vi "Plot Polar Datab.vi"(4 "polar attributes":T3={"maximum"=0.011811645350765643, "minimum"=0.0, "clip to min"=FALSE, "log"=FALSE, "grid color"=6710886, "plot color"=4456703, "fmt and prec"={"format"=enum."Decimal", "precision"=1}, "visible section"=8} {"minimum" format="%.2f"; "maximum" format="%.2f"}, 5 "grid measurements":T2={"pixel center"={"x"=350, "y"=350}, "scale factors"={"a"=28023.191534322883, "b"=0.0, "log?"=FALSE}, "grid color"=6710886, "start angle"=0.0, "end angle"=360.0, "tick length"=333, "pixel radius"=331} {"end angle" format="%.2f"; "start angle" format="%.2f"; "scale factors"."b" format="%.2f"; "scale factors"."a" format="%.2f"}, 6 "polar data":cluster{"magnitude":dbl, "phase":dbl}[](array[cluster])=[{"magnitude"=0.007880735964845577, "phase"=171.85414383638346}, {"magnitude"=0.007585337925796836, "phase"=59.5589656533246}, {"magnitude"=0.009442602002040985, "phase"=266.4429815116384}, {"magnitude"=0.010633627194841278, "phase"=109.76131149110365}, {"magnitude"=0.010068059513029855, "phase"=56.79911977455109}, {"magnitude"=0.009192236833814618, "phase"=70.28455200848899}, {"magnitude"=0.011811645350765643, "phase"=77.24763555601999}, {"magnitude"=0.00992585816138018, "phase"=113.84973004127576}, {"magnitude"=0.008255396341067898, "phase"=111.18742602626722}, {"magnitude"=0.0, "phase"=0.0}] {"phase" format="%.2f"; "magnitude" format="%.2f"}, 7 "picture":picture) -> (3 "new picture":picture)   [LabVIEW 2010]
panel:
  in  "pen":T1={"Width"=6, "Style"=enum."Solid"}
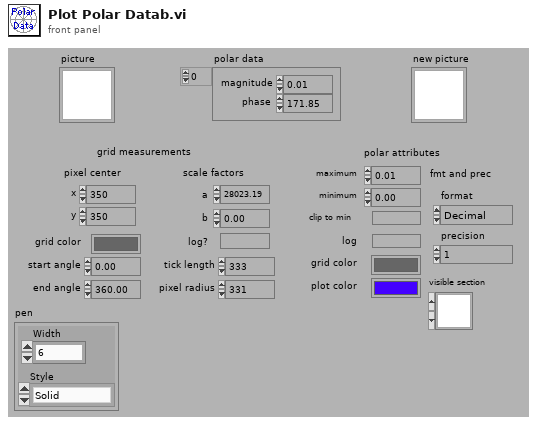
[diagram p1: front panel]
types:
  T1 = cluster{"Width":u16, "Style":enum32{"Solid", "Dash", "Dot", "DashDot", "DashDotDot"}}
  T2 = cluster{"pixel center":cluster{"x":i16, "y":i16}, "scale factors":cluster{"a":dbl, "b":dbl, "log?":bool}, "grid color":u32, "start angle":dbl, "end angle":dbl, "tick length":i16, "pixel radius":i32}
  T3 = cluster{"maximum":dbl, "minimum":dbl, "clip to min":bool, "log":bool, "grid color":u32, "plot color":u32, "fmt and prec":cluster{"format":enum8{"Decimal", "Scientific", "Engineering", "Binary", "Octal", "Hex"}, "precision":u8}, "visible section":u16}
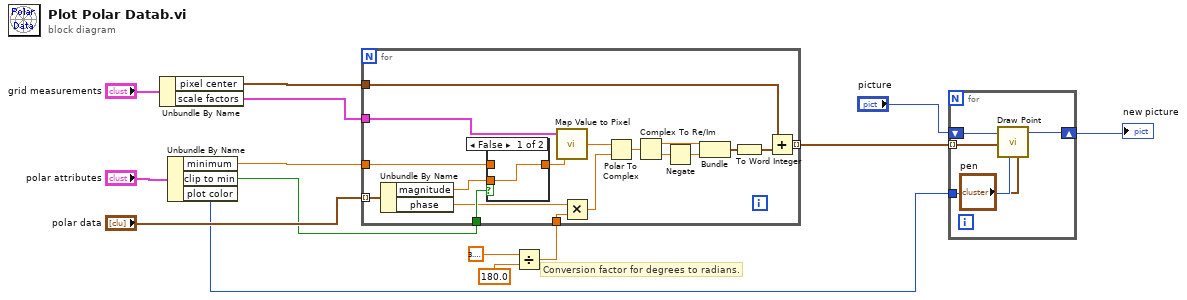
[diagram p0: block diagram]
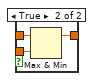
[diagram p2: hidden frame]
diagram:
  # "Conversion factor for degrees to radians."
  n1 = Unbundle By Name("grid measurements") -> ("pixel center"=w10:cluster{"x":i16, "y":i16}, "scale factors"=w11:cluster{"a":dbl, "b":dbl, "log?":bool})
  n2 = Unbundle By Name("polar attributes") -> ("minimum"=w9:dbl, "clip to min"=w8:bool, "plot color"=w2:u32)
  n3 = Divide(x=3.141592653589793, y=180.0) -> (x/y=w6:dbl)
  n4 = for {
    tunnel: "polar data" -> [w32] mode=indexing
    tunnel: w10 -> [w31]
    tunnel: [w30] -> w3 mode=indexing
    tunnel: w11 -> [w23]
    tunnel: w9 -> [w19]
    tunnel: w8 -> [w18]
    tunnel: w6 -> [w15]
    n5 = Unbundle By Name(w32) -> ("magnitude"=w20:dbl, "phase"=w16:dbl)
    n6 = case shown="False" w18 {
      tunnel: w20 -> [w33 w36]
      tunnel: [w33 w35] -> w21
      tunnel: w19 -> [_ w34]
      frame False {
      }
      frame True {
        n7 = Max & Min(x=w34, y=w36) -> (max(x,y)=w35:dbl)  [unwired: 1 out]
      }
    }
    n8 = call <vilib>:"Map Value to Pixel.vi"("x"=w21, "scale factors"=w23) -> ("pixel"=w22:dbl)  [unwired: 1 in]
    n9 = Multiply(x=w16, y=w15) -> (x*y=w17:dbl)
    n10 = Polar To Complex(1:w17, 2:w22) -> (0:w29:cdb)
    n11 = Complex To Re/Im(x + iy=w29) -> (x=w27:dbl, y=w26:dbl)
    n12 = Negate(x=w26) -> (-x=w24:dbl)
    n13 = Bundle(w27, w24) -> (w28:cluster{dbl, dbl})  [unwired: 1 in]
    n14 = To Word Integer(number=w28) -> (16bit integer=w25:cluster{i16, i16})
    n15 = Add(x=w31, y=w25) -> (x+y=w30:cluster{i16, i16})
  }
  n16 = for {
    shift-right: [w41] -> w1
    shift-left: "picture" -> [w38]
    tunnel: w3 -> [w40] mode=indexing
    tunnel: w2 -> [w39]
    n17 = call <vilib>:"Draw Point.vi"("picture"=w38, "point(x,y)"=w40, "color(black)"=w39, "pen"="pen") -> ("new picture"=w41:picture)  [unwired: 5 in]
  }
  "new picture" <- w1
